vi "Cheby derivitaves.vi"(9 "p-the derivative":i32, 10 "Cheby order n":i32, 11 "Coeff":dbl[](array[numeric])=[32.02200051225206, -3.5229923208722456, -0.038405476956685426] format="%.2f") -> (3 "Derivatives":dbl[](array[numeric])=[16.01100025612603, -3.5229923208722456, -0.1536219078267417, 0.0, 0.0])   [LabVIEW 2020]
panel:
  out "T derivatives":dbl[][](array[numeric])=[[0.5, 0.0, 0.0, 0.0, 0.0, 0.0], [0.0, 1.0, 0.0, -3.0, 0.0, 5.0], [0.0, 0.0, 4.0, 0.0, -16.0, 0.0], [0.0, 0.0, 0.0, 24.0, 0.0, -120.0], [0.0, 0.0, 0.0, 0.0, 192.0, 0.0]]
  # "Aij=i th derivative of Tj(x) at x=0\ne.g.  T2(x)=2x^2-1, T2(x)'=4x, T2(x)\"=4\nA12: 1st derivative of T2'(0) = 0\nA22=T2''(0)=4"
  # "A00 is modified to take care of the additional constant term."
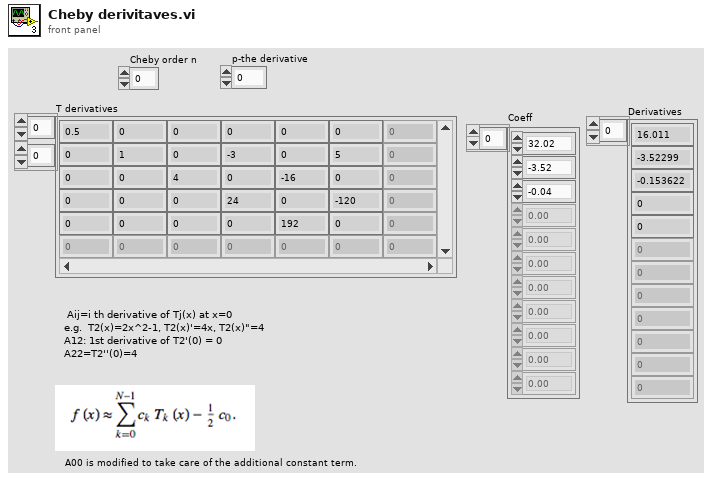
[diagram p1: front panel]
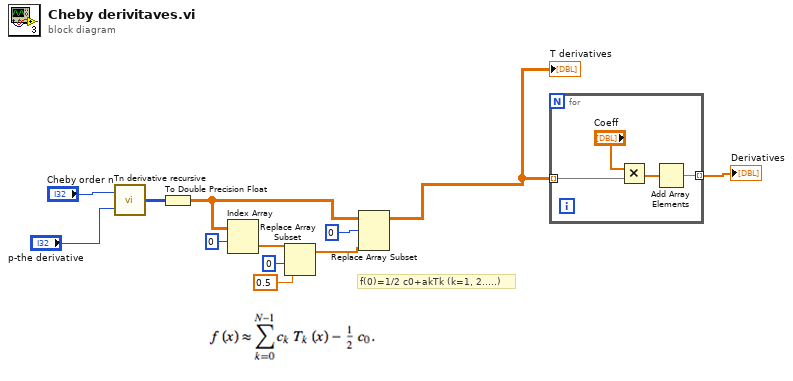
[diagram p0: block diagram]
diagram:
  # "f(0)=1/2 c0+akTk (k=1, 2.....)"
  n1 = call "Tn derivative recursive.vi"("p-the derivative"="p-the derivative", "n"="Cheby order n") -> ("Tn^p (0) array"=w9:i32[][])
  n2 = To Double Precision Float(number=w9) -> (double precision float=w4:dbl[][])
  n3 = Index Array(array=w4, index (row)=0) -> (element=w7:dbl[])  [unwired: 1 in]
  n4 = Replace Array Subset(array=w7, new element=0.5 ("new element/subarray"), index=0) -> (w2:dbl[])
  n5 = Replace Array Subset(array=w4, new element=w2, index (row)=0) -> (w1:dbl[][])  [unwired: 1 in]
  "T derivatives" <- w1
  n6 = for {
    tunnel: w1 -> [w16] mode=indexing
    tunnel: [w14] -> w12 mode=indexing
    n7 = Multiply(x="Coeff", y=w16) -> (x*y=w15:dbl[])
    n8 = Add Array Elements(numeric array=w15) -> (sum=w14:dbl)
  }
  "Derivatives" <- w12
